vi "Parse Record Values.vi"(8 "error in":errorcluster, 9 "End Time":timestamp, 10 "Start Time":timestamp, 11 "Record Values":string[](array[string])) -> (0 "error out":errorcluster, 2 "Raw Data":dbl[][](array[numeric]), 3 "Resampled Data":waveform(dbl))   [LabVIEW 2013, in "Data Log Fetcher.lvlib"]
uses:
  Data Log Fetcher.lvlib
panel:
  out "Sorted Entries":string[](array[string])
  out "Waveform Graph":dbl[](graph)
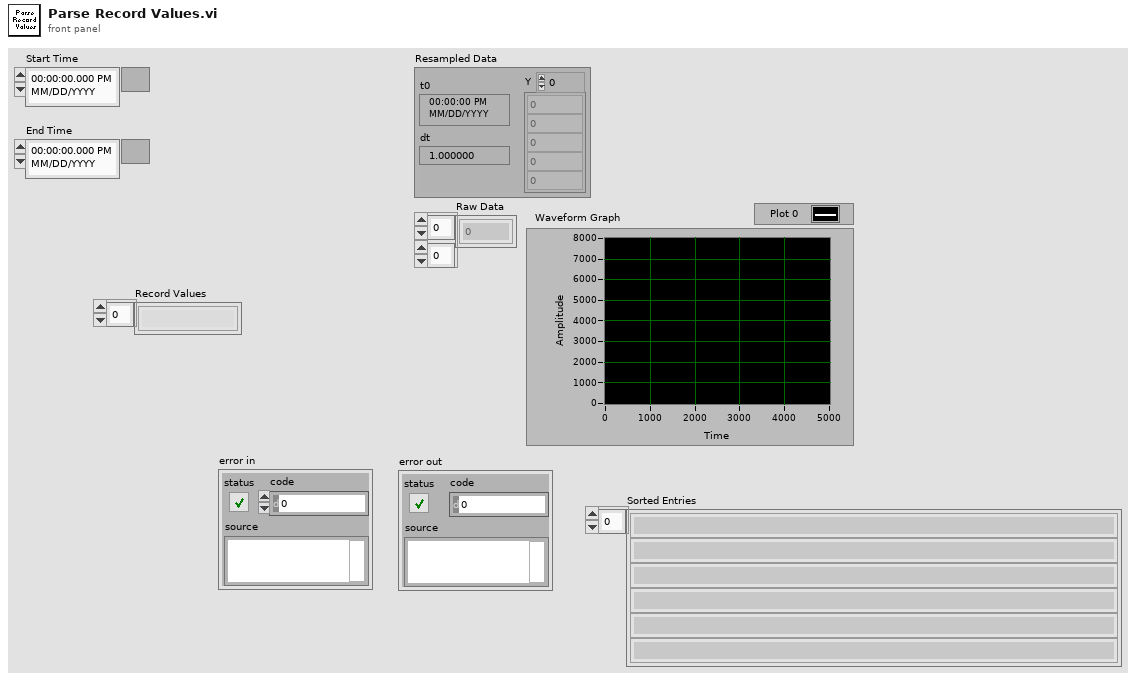
[diagram p1: front panel]
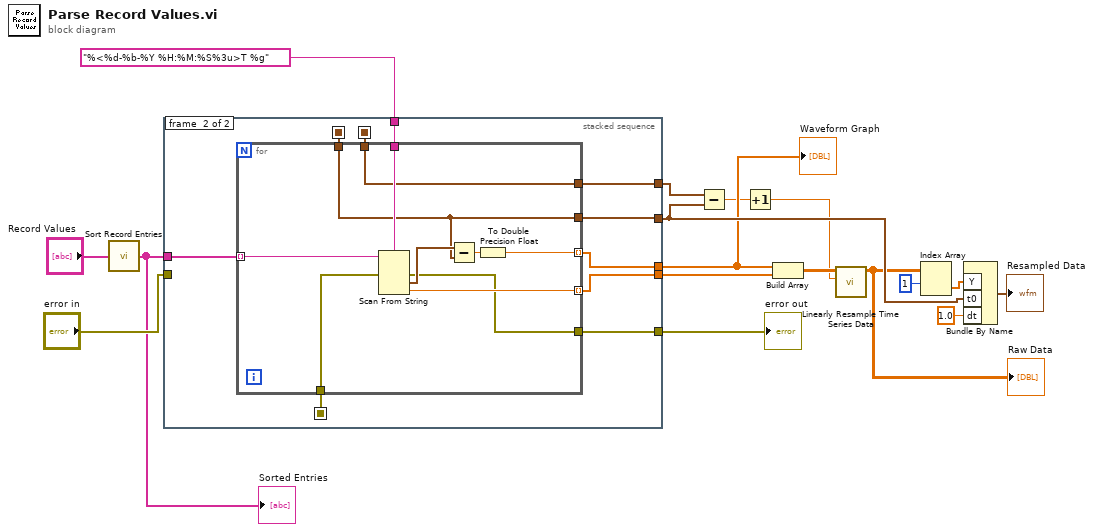
[diagram p0: block diagram]
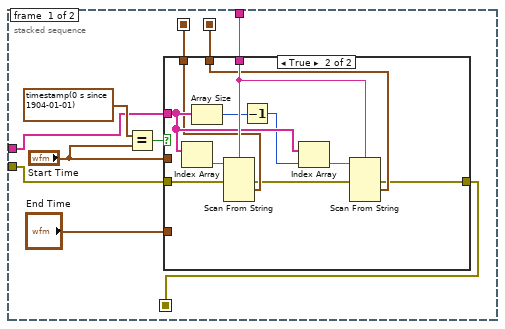
[diagram p2: hidden frame]
diagram:
  n1 = call "Sort Record Entries.vi"("Entries"="Record Values") -> ("Sorted Entries"=w5:string[])  [unwired: 4 in]
  "Sorted Entries" <- w5
  n2 = stacked-sequence {
    seq-local: [w21 _] -> [_ w45]
    seq-local: [w20 _] -> [_ w44]
    seq-local: [w18 _] -> [_ w42]
    tunnel: "%<%d-%b-%Y %H:%M:%S%3u>T %g" ("format string") -> [w23 w51]
    tunnel: [_ w50] -> w14
    tunnel: [_ w49] -> w3
    tunnel: [_ w48] -> w13
    tunnel: "error in" -> [w19 _]
    tunnel: [_ w47] -> w7
    tunnel: w5 -> [w22 w46]
    tunnel: [_ w43] -> w4
    frame #0 {
      n3 = Equal?(x=timestamp(0 s since 1904-01-01) ("Start Time"), y="Start Time") -> (x = y?=w26:bool)
      n4 = case shown="True" w26 {
        tunnel: "Start Time" -> [w30 _]
        tunnel: "End Time" -> [w29 _]
        tunnel: w23 -> [_ w41]
        tunnel: w22 -> [_ w37]
        tunnel: [w30 w35] -> w21
        tunnel: [w29 w34] -> w20
        tunnel: w19 -> [w28 w33]
        tunnel: [w28 w31] -> w18
        frame False {
        }
        frame True {
          n5 = Index Array(array=w37) -> (element=w40:string)  [unwired: 1 in]
          n6 = Array Size(array=w37) -> (size(s)=w39:i32)
          n7 = Scan From String(format string=w41, input string=w40, error in=w33) -> (error out=w32:errorcluster, output 1=w35:timestamp)  [unwired: 4 in, 2 out]
          n8 = Decrement(x=w39) -> (x-1=w36:i32)
          n9 = Index Array(array=w37, index=w36) -> (element=w38:string)
          n10 = Scan From String(format string=w41, input string=w38, error in=w32) -> (error out=w31:errorcluster, output 1=w34:timestamp)  [unwired: 4 in, 2 out]
        }
      }
    }
    frame #1 {
      n11 = for {
        tunnel: w51 -> [w61]
        tunnel: w46 -> [w58] mode=indexing
        tunnel: [w54] -> w50
        tunnel: [w57] -> w49 mode=indexing
        tunnel: [w56] -> w48 mode=indexing
        tunnel: [w55] -> w47
        tunnel: w45 -> [w54]
        tunnel: [w53] -> w43
        tunnel: w44 -> [w53]
        tunnel: w42 -> [w52]
        n12 = Scan From String(format string=w61, input string=w58, error in=w52) -> (error out=w55:errorcluster, output 1=w59:timestamp, output 2=w56:dbl)  [unwired: 3 in, 2 out]
        n13 = Subtract(x=w59, y=w54) -> (x-y=w60:dbl)
        n14 = To Double Precision Float(number=w60) -> (double precision float=w57:dbl)
      }
    }
  }
  "error out" <- w7
  "Waveform Graph" <- w3
  n15 = Subtract(x=w4, y=w14) -> (x-y=w2:dbl)
  n16 = Increment(x=w2) -> (x+1=w1:dbl)
  n17 = Build Array(w3, w13) -> (w12:dbl[][])
  n18 = call "Linearly Resample Time Series Data.vi"("Duration (s)"=w1, "Irregular Data"=w12) -> ("Regular Data"=w11:dbl[][])  [unwired: 9 in]
  "Raw Data" <- w11
  n19 = Index Array(array=w11, index (row)=1) -> (element=w10:dbl[])  [unwired: 1 in]
  n20 = Bundle By Name("Y"=w10, "t0"=w14, "dt"=1.0) -> (→"Resampled Data":waveform(dbl))  [unwired: 1 in]
